vi "error case.vi"() -> ()   [LabVIEW 2013]
panel:
  in  "error in":errorcluster
  out "error out":errorcluster
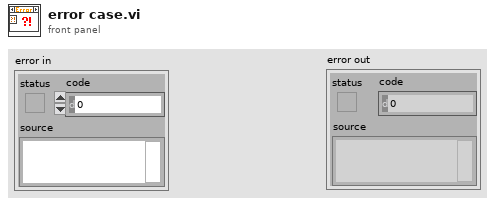
[diagram p1: front panel]
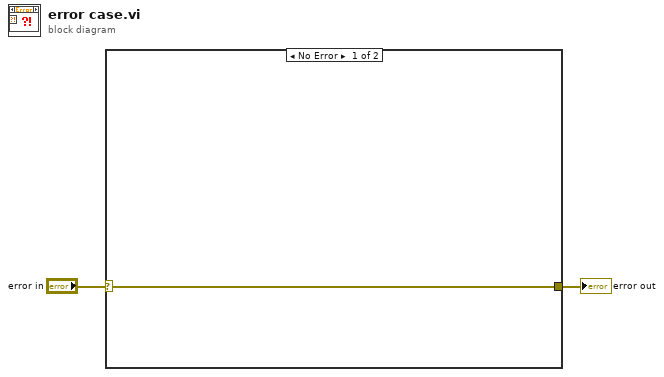
[diagram p0: block diagram]
diagram:
  n1 = case shown="No Error" "error in" {
    selector: "error in" -> [w3 w4]
    tunnel: [w3 w4] -> w2
    frame No Error {
    }
    frame Error {
    }
  }
  "error out" <- w2
